vi "UnboxVariant.vi"(10 "Variant In":refnum<class "Variant.lvclass">) -> (2 "Variant":variant)   [LabVIEW 2013, in "LapDog.Collections.v1.Common.lvlib" / "Variant.lvclass"]
uses:
  Variant.lvclass
  Variant.lvclass/Variant.ctl
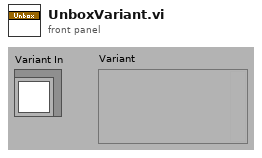
[diagram p1: front panel]
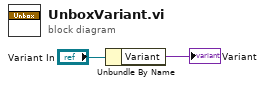
[diagram p0: block diagram]
diagram:
  n1 = Unbundle By Name("Variant In") -> ("Variant"=→"Variant":variant)
